vi "Get Active Bool Function.vi"(0 "Boolean Functions in":refnum<class "Boolean Functions.lvclass">, 11 "error in (no error)":errorcluster) -> (4 "Boolean Functions out":refnum<class "Boolean Functions.lvclass">, 6 "Function":T1, 15 "error out":errorcluster)   [LabVIEW 2019, in "Boolean Functions.lvclass"]
uses:
  Boolean Functions.lvclass
  D:/Pet Projects/LSL/source code/LSL components/functions/functionsbase/functionbase.lvclass
  Function List.ctl
  functionsbase/functionbase.lvclass
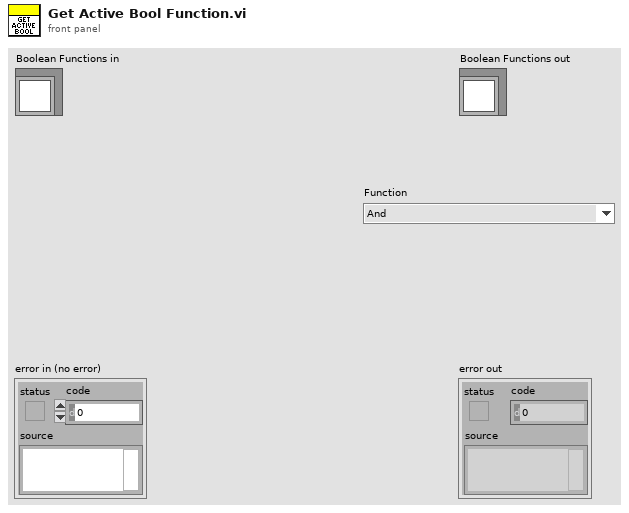
[diagram p1: front panel]
types:
  T1 = typedef "Boolean Functions.lvclass/Function List.ctl" = enum16{"And", "Or", "Exclusive Or", "Not", "Not And", "Not Or", "Not Exclusive Or", "Random Bool"}
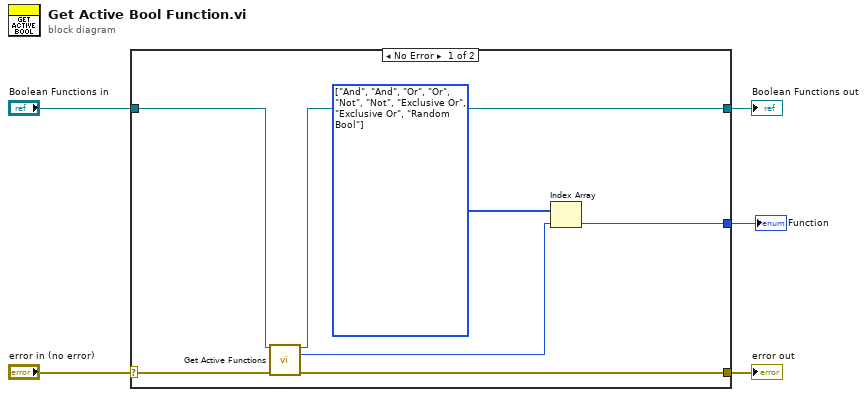
[diagram p0: block diagram]
diagram:
  n1 = case shown="No Error" "error in (no error)" {
    selector: "error in (no error)" -> [w12 w14]
    tunnel: [w11 w14] -> w4
    tunnel: [w9 w13] -> w2
    tunnel: "Boolean Functions in" -> [w10 w13]
    tunnel: [w6 _] -> w1
    frame No Error {
      w8 = T1[] [enum."And", enum."And", enum."Or", enum."Or", enum."Not", enum."Not", enum."Exclusive Or", enum."Exclusive Or", enum."Random Bool"] items=["And", "Or", "Exclusive Or", "Not", "Not And", "Not Or", "Not Exclusive Or", "Random Bool"]
      n2 = call "Get Active Functions.vi"("functionbase in"=w10, "error in (no error)"=w12) -> ("functionbase out"=w9:refnum<class "Boolean Functions.lvclass">, "Syntax Index"=w7:i32, "error out"=w11:errorcluster)  [unwired: 11 in]
      n3 = Index Array(array=w8, index=w7) -> (element=w6:T1)
    }
    frame Error {
    }
  }
  "error out" <- w4
  "Boolean Functions out" <- w2
  "Function" <- w1
